vi "TPNT_ParseAlarmField.vi"(11 "Alarm Field":string) -> (0 "after":i32, 1 "every msecs":bool, 2 "every":i32, 3 "action":string, 4 "max":i32)   [LabVIEW 2016]
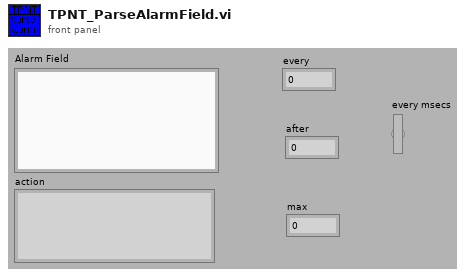
[diagram p1: front panel]
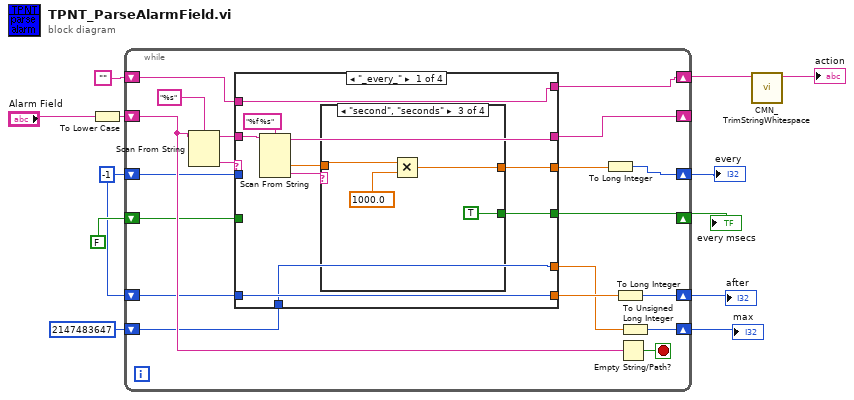
[diagram p0: block diagram]
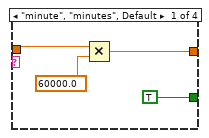
[diagram p2: hidden frame]
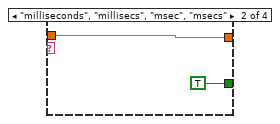
[diagram p3: hidden frame]
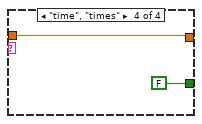
[diagram p4: hidden frame]
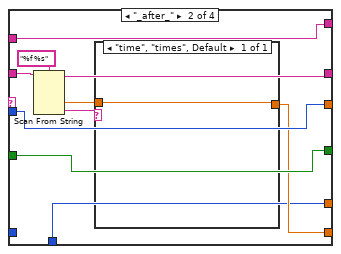
[diagram p5: hidden frame]
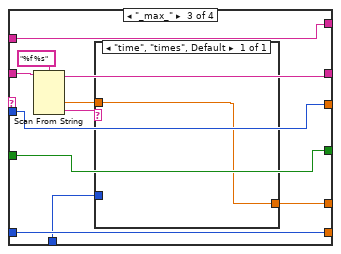
[diagram p6: hidden frame]
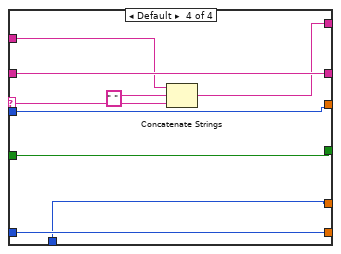
[diagram p7: hidden frame]
diagram:
  w2 = -1
  n1 = To Lower Case(string="Alarm Field") -> (all lower case string=w11:string)
  n2 = while {
    shift-right: [w26] -> _
    shift-left: w11 -> [w28]
    shift-right: [w24] -> w10
    shift-left: w2 -> [w21]
    shift-right: [w23] -> w9
    shift-left: FALSE -> [w22]
    shift-right: [w18] -> w8
    shift-left: w2 -> [w20]
    shift-right: [w16] -> w5
    shift-left: "" -> [w17]
    shift-right: [w13] -> w3
    shift-left: 2147483647 -> [w15]
    stop <- w27 stop-if-true
    n3 = Scan From String(format string="%s", input string=w28) -> (remaining string=w29:string, output 1=w30:string)  [unwired: 2 in, 3 out]
    n4 = case shown="\"_every_\"" w30 {
      selector: w30 -> [_ _ _ w78]
      tunnel: [w39 w61 w73 w85] -> w26
      tunnel: w29 -> [w41 w63 w75 w85]
      tunnel: [w36 w58 w70 w83] -> w25
      tunnel: [w35 w57 w69 w84] -> w23
      tunnel: w22 -> [_ w57 w69 w84]
      tunnel: w21 -> [_ w58 w70 w83]
      tunnel: w20 -> [w34 _ w67 w82]
      tunnel: [w34 w56 w67 w82] -> w19
      tunnel: w17 -> [w33 w55 w68 w81]
      tunnel: [w33 w55 w68 w80] -> w16
      tunnel: w15 -> [w32 w54 w66 w77]
      tunnel: [w32 w54 w65 w77] -> w14
      frame "_every_" {
        n5 = Scan From String(format string="%f %s", input string=w41) -> (remaining string=w39:string, output 1=w37:dbl, output 2=w38:string)  [unwired: 2 in, 4 out]
        n6 = case shown="\"second\", \"seconds\"" w38 {
          tunnel: w37 -> [w45 w47 w51 w53]
          tunnel: [w43 w47 w49 w53] -> w36
          tunnel: [TRUE TRUE TRUE FALSE] -> w35
          frame "minute", "minutes", Default {
            n7 = Multiply(x=w45, y=60000.0) -> (x*y=w43:dbl)
          }
          frame "milliseconds", "millisecs", "msec", "msecs" {
          }
          frame "second", "seconds" {
            n8 = Multiply(x=w51, y=1000.0) -> (x*y=w49:dbl)
          }
          frame "time", "times" {
          }
        }
      }
      frame "_after_" {
        n9 = Scan From String(format string="%f %s", input string=w63) -> (remaining string=w61:string, output 1=w59:dbl, output 2=w60:string)  [unwired: 2 in, 4 out]
        n10 = case shown="\"time\", \"times\", Default" w60 {
          tunnel: w59 -> [w64]
          tunnel: [w64] -> w56
          frame "time", "times", Default {
          }
        }
      }
      frame "_max_" {
        n11 = Scan From String(format string="%f %s", input string=w75) -> (remaining string=w73:string, output 1=w71:dbl, output 2=w72:string)  [unwired: 2 in, 4 out]
        n12 = case shown="\"time\", \"times\", Default" w72 {
          tunnel: w71 -> [w76]
          tunnel: w66 -> [_]
          tunnel: [w76] -> w65
          frame "time", "times", Default {
          }
        }
      }
      frame Default {
        n13 = Concatenate Strings(w81, " ", w78) -> (w80:string)
      }
    }
    n14 = To Long Integer(number=w25) -> (32bit integer=w24:i32)
    n15 = To Long Integer(number=w19) -> (32bit integer=w18:i32)
    n16 = Empty String/Path?(string/path=w28) -> (empty?=w27:bool)
    n17 = To Unsigned Long Integer(number=w14) -> (unsigned 32bit integer=w13:u32)
  }
  "after" <- w8
  "every" <- w10
  "every msecs" <- w9
  "max" <- w3
  n18 = call "CMN_TrimStringWhitespace.vi"("string"=w5) -> ("trimmed string"=→"action":string)  [unwired: 1 in, 8 out]
